vi "Update path [ ].vi"(1 "Support Directory Name (EXE)":string="Data", 3 "Image to Add IN [ ]":T2(array[cluster]) {"Scale" format="%#_g %"}) -> (0 "Image to Add OUT [ ]":T2(array[cluster]) {"Scale" format="%#_g %"})   [LabVIEW 2019]
doc: "Update the path for different versions of LV."
uses:
  <userlib>/Exaprom PDF/Controls/Image Controls/Image Scale.ctl
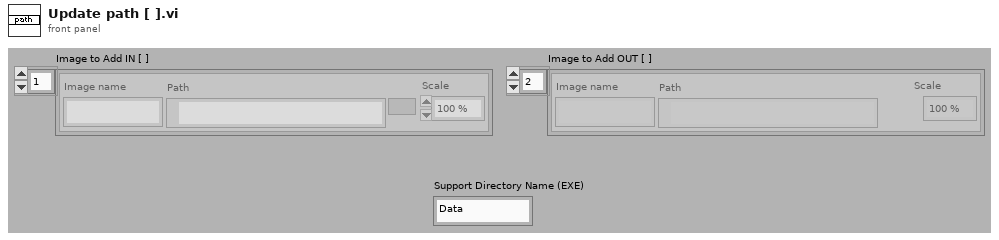
[diagram p1: front panel]
types:
  T1 = typedef "Image Scale.ctl" = sgl
  T2 = cluster{"Image name":string, "Path":path, "Scale":T1}[]
  T3 = cluster{"Image name":string, "Path":path, "Scale":T1}
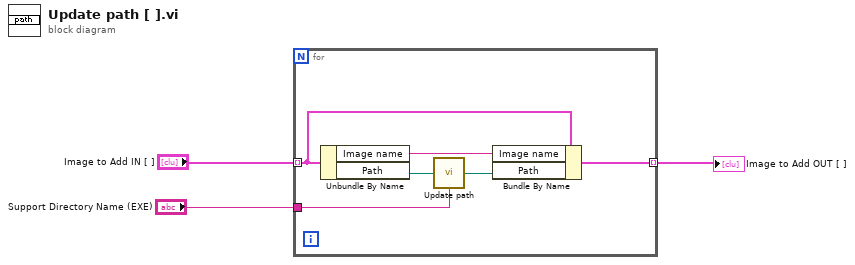
[diagram p0: block diagram]
diagram:
  n1 = for {
    tunnel: "Image to Add IN [ ]" -> [w9] mode=indexing
    tunnel: [w8] -> w2 mode=indexing
    tunnel: "Support Directory Name (EXE)" -> [w4]
    n2 = Unbundle By Name(w9) -> ("Image name"=w7:string, "Path"=w6:path)
    n3 = call <userlib>:"Update path.vi"("Support Directory Name (EXE)"=w4, "Path IN"=w6) -> ("Path OUT"=w5:path)  [unwired: 2 in]
    n4 = Bundle By Name(cluster=w9, "Image name"=w7, "Path"=w5) -> (w8:T3)
  }
  "Image to Add OUT [ ]" <- w2
